vi "Denoising with Wavelet (Measurements).vi"() -> ()   [LabVIEW 2023]
doc: "This example shows how to reduce noise of an image with the WA Denoise VI. The flower image is contaminated by some Gaussian white noise with a standard deviation 5. This example uses the undecimated wavelet transform-based method to denoise the image.\n\n<b>Instructions:</b>\n1) Run this VI.\n2) Compare the noisy image and denoised image with different settings."
uses:
  Images/_Images.ctl
  <vilib>/addons/Wavelet Analysis/application.llb/WA Denoise (UWT 2D Array).vi
  <vilib>/addons/_Advanced Signal Processing/NI_AdvSigProcWA.lvlib
  <vilib>/vision/NI_Vision_Development_Module.lvlib
panel:
  out "CNR Thick 2":dbl
  out "CNR Thin 2":dbl
  out "SNR Thick 2":sgl format="%.2f"
  out "SNR Thin 2":sgl format="%.2f"
  out "CNR Thick":dbl
  out "CNR Thin":dbl
  out "SNR Thick":sgl format="%.2f"
  out "SNR Thin":sgl format="%.2f"
  out "Crop":T1(plugin-control)
  out "Crop":T1(plugin-control)
  out "Denoised Image":T1(plugin-control)
  out "Image Src":T1(plugin-control)
  in  "Threshold settings":T2={"Thresholding Rule"=enum."SURE", "Rescaling Method"=enum."Single level", "Soft Threshold?"=TRUE}
  in  "Wavelet":u16(ring) items=["db02"=0, "db03"=1, "db04"=2, "db05"=3, "db06"=4, "db07"=5, "db08"=6, "db09"=7, "db10"=8, "db11"=9, "db12"=10, "db13"=11, "db14"=12, "Haar"=13, "bior1_3"=14, "bior1_5"=15, "bior2_2"=16, "bior2_4"=17, "bior2_6"=18, "bior2_8"=19, "bior3_1"=20, "bior3_3"=21, "bior3_5"=22, "bior3_7"=23, "bior3_9"=24, "bior4_4 (FBI)"=25, "bior5_5"=38, "bior6_8"=39, "coif1"=26, "coif2"=27, "coif3"=28, "coif4"=29, "coif5"=30, "sym2"=31, "sym3"=32, "sym4"=33, "sym5"=34, "sym6"=35, "sym7"=36, "sym8"=37]
  in  "Levels":i32=4
  # "Images Denoising\nusing Wavelets"
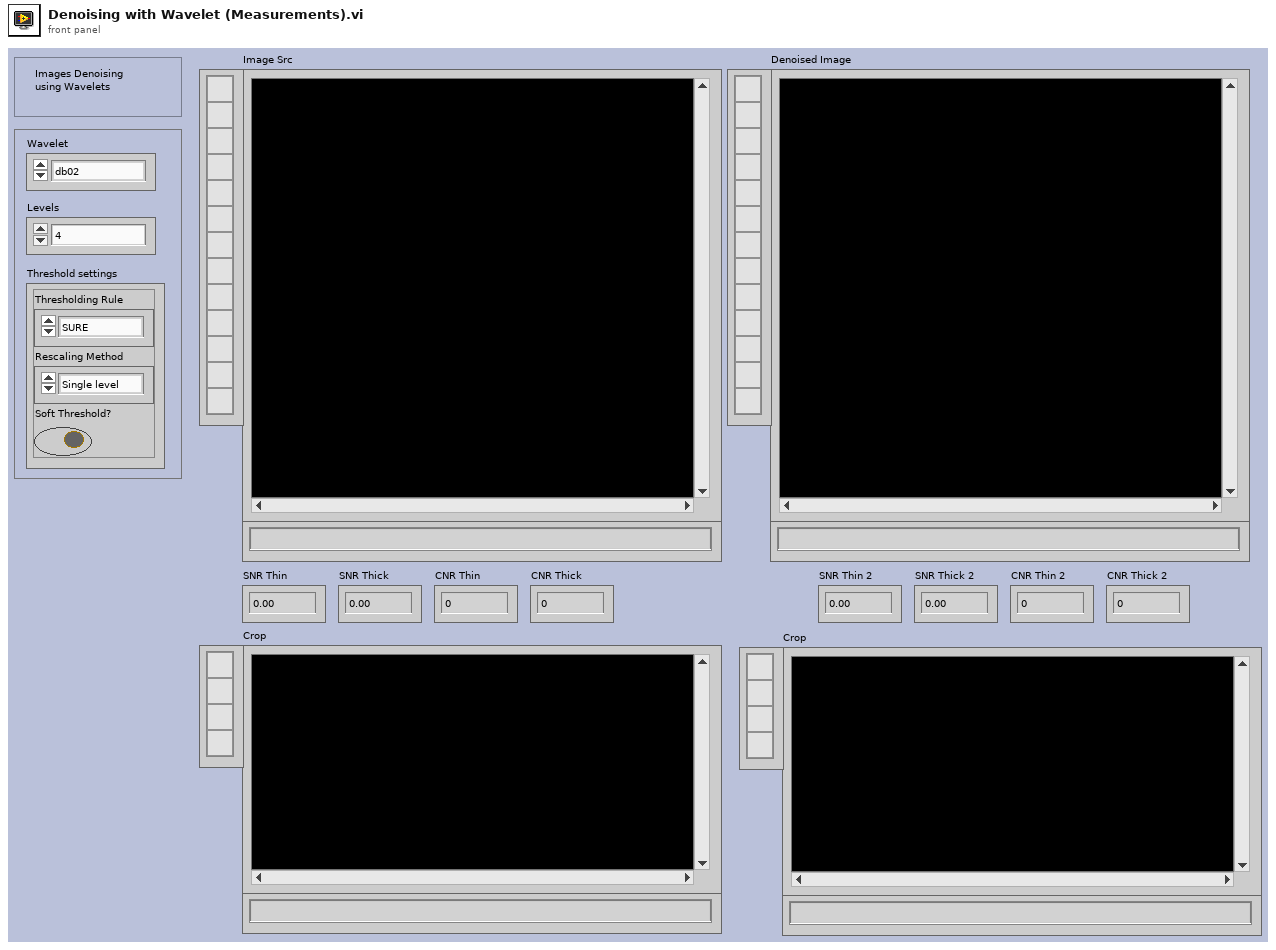
[diagram p1: front panel]
types:
  T1 = typedef "IMAQ Image.ctl" = refnum<image>
  T2 = cluster{"Thresholding Rule":enum16{"SURE", "Hybrid", "Universal", "Minimax"}, "Rescaling Method":enum16{"One", "Single level", "Multiple levels"}, "Soft Threshold?":bool}
  T3 = cluster{"Global Rectangle":i32[], "Contours":cluster{"Contour Type":u32, "ROI Type":u32, "Points":i32[]}[]}
  T4 = typedef "IMAQ Point" = cluster{"X":sgl, "Y":sgl}
  T5 = typedef "Image Type" = u32
  T6 = typedef "_Images.ctl" = enum16{"Ostern2023", "Balls2", "Battery1", "Battery2", "Connector1", "Subwoofer1", "Subwoofer2", "Subwoofer3", "Subwoofer4", "Hase1", "Lamp1", "Lamp2", "Mouse1", "PhotoLens1", "Po1", "PowerSupply1", "Router", "--- Step Wedges ---", "Stepwedge1", "Stepwedge2", "Stepwedge3", "--- Fusion ---", "Fusion160kV", "Fusion2-120kV", "Fusion2-320kV", "Fusion300kV", "FusionPart1-120kV", "FusionPart1-180kV", "--- PART 01 ---", "Part1", "Part2", "Part3", "Part4", "Part5", "Part6", "Part7", "Part8", "--- Different Integrations ---", "Step2737-02Int", "Step2737-04Int", "Step2737-08Int", "Step2737-16Int", "Step2737-32Int", "Step2737-64Int"}
  T7 = cluster{"SNR Thin":sgl, "SNR Thick":sgl, "Signal Level Thin":sgl, "Signal Level Thick":sgl, "SNRn Thin":sgl, "SNRn Thick":sgl}
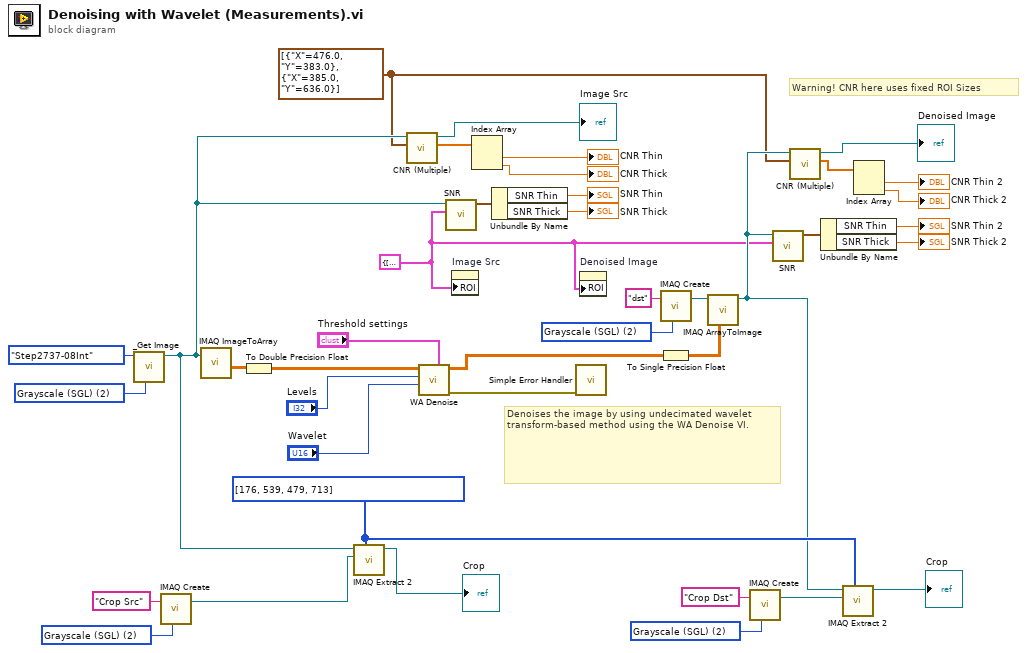
[diagram p0: block diagram]
diagram:
  w3 = T3 {"Global Rectangle"=[47, 353, 968, 848], "Contours"=[{"Contour Type"=0, "ROI Type"=3, "Points"=[100, 350, 150, 400]}, {"Contour Type"=0, "ROI Type"=3, "Points"=[850, 350, 900, 400]}, {"Contour Type"=0, "ROI Type"=3, "Points"=[100, 700, 150, 750]}, {"Contour Type"=0, "ROI Type"=3, "Points"=[850, 700, 900, 750]}]} ("ROI")
  w4 = T4[] [{"X"=476.0, "Y"=383.0}, {"X"=385.0, "Y"=636.0}]
  w21 = i32[] [176, 539, 479, 713] ("appended array")
  w27 = T5 2 items=["Grayscale (U8)", "Grayscale (I16)", "Grayscale (SGL)", "Complex (CSG)", "RGB (U32)", "HSL (U32)", "RGB (U64)", "Grayscale (U16)"] ("Image Type")
  w22 = T5 2 items=["Grayscale (U8)", "Grayscale (I16)", "Grayscale (SGL)", "Complex (CSG)", "RGB (U32)", "HSL (U32)", "RGB (U64)", "Grayscale (U16)"] ("Image Type")
  w29 = T5 2 items=["Grayscale (U8)", "Grayscale (I16)", "Grayscale (SGL)", "Complex (CSG)", "RGB (U32)", "HSL (U32)", "RGB (U64)", "Grayscale (U16)"] ("Image Type")
  w34 = T5 2 items=["Grayscale (U8)", "Grayscale (I16)", "Grayscale (SGL)", "Complex (CSG)", "RGB (U32)", "HSL (U32)", "RGB (U64)", "Grayscale (U16)"] ("Image Type (U16)")
  # "Warning! CNR here uses fixed ROI Sizes"
  # "Denoises the image by using undecimated wavelet transform-based method using the WA Denoise VI."
  n1 = call "_Get Image.vi"("Image Type (U16)"=w34, "Image"=_Images."Step2737-08Int") -> ("Image Out"=w14:T1)  [unwired: 6 in, 3 out]
  n2 = call "IMAQ Create"("Image Name"="Crop Src", "Image Type"=w22) -> ("New Image"=w24:T1)  [unwired: 3 in, 1 out]
  n3 = call "IMAQ ImageToArray"("Image"=w14) -> ("Image Pixels (Float)"=w33:sgl[][])  [unwired: 3 in, 4 out]
  n4 = To Double Precision Float(number=w33) -> (double precision float=w36:dbl[][])
  n5 = call "IMAQ Extract 2"("Optional Rectangle"=w21, "Image Dst"=w24, "Image Src"=w14) -> ("Image Dst Out"=→"Crop":T1)  [unwired: 7 in, 1 out]
  n6 = call "CNR (Multiple).vi"("Array of the Points\nfor Measurement"=w4, "Refnum in"=w14) -> ("Array out"=w12:dbl[], "Refnum out"=→"Image Src":T1)  [unwired: 8 in]
  n7 = call-poly <vilib>:"WA Denoise.vi"("threshold settings"="Threshold settings", "wavelet"="Wavelet", "levels"="Levels", "signal"=w36) -> ("error out"=w37:errorcluster, "denoised signal"=w31:dbl[][])  [unwired: 1 in, 5 out]
  n8 = call "SNR.vi"("ROI"=w3, "Refnum in"=w14) -> ("SNR Results"=w20:T7)  [unwired: 9 in]
  n9 = property on="Image Src" class="ImageControl"("ROI"=w3) -> ()  [unwired: 2 in, 2 out]
  n10 = Index Array(array=w12) -> (element #1=→"CNR Thin":dbl, element #2=→"CNR Thick":dbl)  [unwired: 2 in]
  n11 = Unbundle By Name(w20) -> ("SNR Thin"=→"SNR Thin":sgl, "SNR Thick"=→"SNR Thick":sgl)
  n12 = call <vilib>:"Simple Error Handler.vi"("error in (no error)"=w37) -> ()  [unwired: 4 in, 5 out]
  n13 = property on="Denoised Image" class="ImageControl"("ROI"=w3) -> ()  [unwired: 2 in, 2 out]
  n14 = call "IMAQ Create"("Image Name"="dst", "Image Type"=w29) -> ("New Image"=w30:T1)  [unwired: 3 in, 1 out]
  n15 = To Single Precision Float(number=w31) -> (single precision float=w28:sgl[][])
  n16 = call "IMAQ ArrayToImage"("Image Pixels (Float)"=w28, "Image"=w30) -> ("Image Out"=w9:T1)  [unwired: 8 in, 1 out]
  n17 = call "IMAQ Create"("Image Name"="Crop Dst", "Image Type"=w27) -> ("New Image"=w25:T1)  [unwired: 3 in, 1 out]
  n18 = call "SNR.vi"("ROI"=w3, "Refnum in"=w9) -> ("SNR Results"=w17:T7)  [unwired: 9 in]
  n19 = call "CNR (Multiple).vi"("Array of the Points\nfor Measurement"=w4, "Refnum in"=w9) -> ("Array out"=w7:dbl[], "Refnum out"=→"Denoised Image":T1)  [unwired: 8 in]
  n20 = Unbundle By Name(w17) -> ("SNR Thin"=→"SNR Thin 2":sgl, "SNR Thick"=→"SNR Thick 2":sgl)
  n21 = call "IMAQ Extract 2"("Optional Rectangle"=w21, "Image Dst"=w25, "Image Src"=w9) -> ("Image Dst Out"=→"Crop":T1)  [unwired: 7 in, 1 out]
  n22 = Index Array(array=w7) -> (element #1=→"CNR Thin 2":dbl, element #2=→"CNR Thick 2":dbl)  [unwired: 2 in]
